vi "Append Suffix to VI Name.vi"(8 "error in (no error)":errorcluster, 10 "VI Title Suffix":string, 11 "VI in":refnum<vi>) -> (0 "Error Out":errorcluster)   [LabVIEW 2021, in "GUI.lvlib"]
uses:
  GUI.lvlib
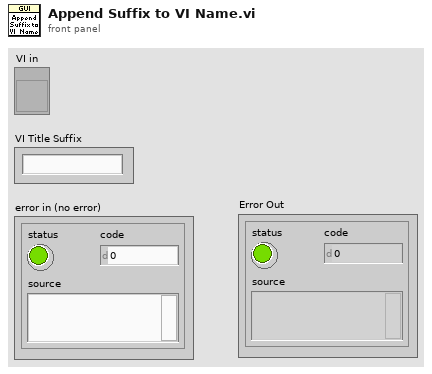
[diagram p1: front panel]
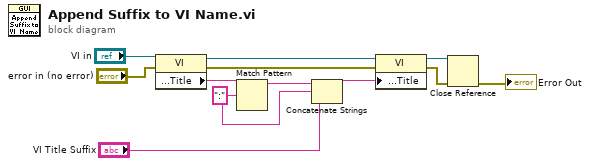
[diagram p0: block diagram]
diagram:
  w3 = ":" ("regular expression")
  n1 = property class="VI"(reference="VI in", error in="error in (no error)") -> (reference out=w6:refnum<vi>, error out=w1:errorcluster, "Front Panel.Title"=w5:string)
  n2 = Match Pattern(string=w5, regular expression=w3) -> (before substring=w4:string)  [unwired: 1 in, 3 out]
  n3 = Concatenate Strings(w4, w3, "VI Title Suffix") -> (w11:string)
  n4 = property class="VI"(reference=w6, error in=w1, "Front Panel.Title"=w11) -> (reference out=w10:refnum<vi>, error out=w9:errorcluster)
  n5 = Close Reference(reference=w10, error in (no error)=w9) -> (error out=→"Error Out":errorcluster)
